vi "table line to eiptag.vi"(11 "line strings":string[](array[string])) -> (2 "invalid?":bool, 3 "tag":T1={"eip tag types"=enum."SINT", "unique tag name"="", "Number of Elements"=1})   [LabVIEW 2013, in "EIP Tags editor node.lvclass"]
uses:
  EIP Tags editor node.lvclass
  <vilib>/NI/TBM Modules/EIP Tags/configuration/eip tag definition.ctl
  <vilib>/NI/TBM Modules/EIP Tags/configuration/eip tag types.ctl
  <vilib>/NI/TBM Modules/EIP Tags/configuration/EIP Tags Configuration.lvclass
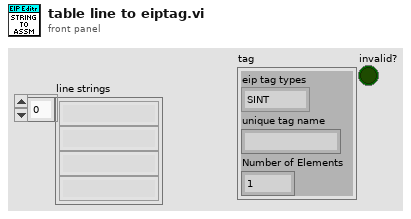
[diagram p1: front panel]
types:
  T1 = typedef "EIP Tags Configuration.lvclass/eip tag definition.ctl" = cluster{"eip tag types":T2, "unique tag name":string, "Number of Elements":u32}
  T2 = typedef "EIP Tags Configuration.lvclass/eip tag types.ctl" = enum16{"SINT", "INT", "DINT", "REAL", "BOOL", "STRING"}
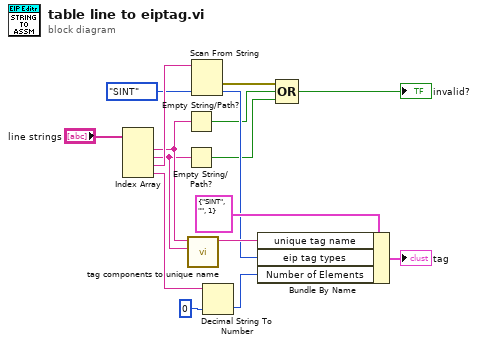
[diagram p0: block diagram]
diagram:
  n1 = Index Array(array="line strings") -> (element #1=w6:string, element #2=w5:string, element #3=w9:string, element #4=w12:string)  [unwired: 4 in]
  n2 = Empty String/Path?(string/path=w6) -> (empty?=w3:bool)
  n3 = Empty String/Path?(string/path=w5) -> (empty?=w4:bool)
  n4 = call <vilib>:"tag components to unique name.vi"("Tag Name"=w5, "Network Path"=w6) -> ("unique name"=w13:string)  [unwired: 9 in]
  n5 = Scan From String(input string=w9, default 1=eip_tag_types."SINT" ("eip tag types")) -> (error out=w2:errorcluster, output 1=w7:T2)  [unwired: 3 in, 2 out]
  n6 = Decimal String To Number(string=w12, default (0L)=u32 0 ("default (0 I32)")) -> (number=w11:u32)  [unwired: 1 in, 1 out]
  n7 = Bundle By Name(cluster=T1 {"eip tag types"=enum."SINT", "unique tag name"="", "Number of Elements"=1} ("tag spec"), "unique tag name"=w13, "eip tag types"=w7, "Number of Elements"=w11) -> (→"tag":T1)
  n8 = Compound Arithmetic op=OR(w2, w3, w4) -> (→"invalid?":bool)
